vi "Add setting.vi"(7 "setting reference":refnum<vi>, 8 "error in (no error)":errorcluster, 11 "ServiceManager in":refnum<class "ServiceManager.lvclass">) -> (0 "error out":errorcluster, 3 "ServiceManager out":refnum<class "ServiceManager.lvclass">)   [LabVIEW 2012, in "ServiceManager.lvclass"]
uses:
  ServiceManager.lvclass
  settings_cluster.ctl
  Murmex/LabVIEW/Murmex/Murmex/component_specification_cluster.ctl
  ServiceManager.lvclass/ServiceManager.ctl
  Murmex/LabVIEW/Murmex/Murmex/Murmex.lvclass
panel:
  in  "button:cancel":bool
  in  "button:confirm":bool
  in  "Name":string
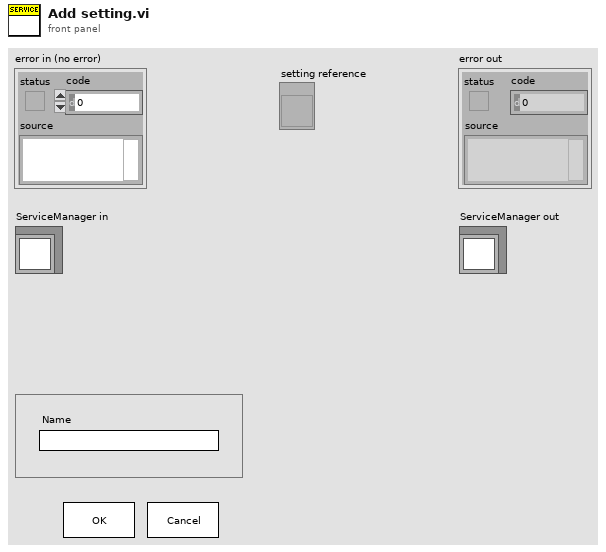
[diagram p1: front panel]
types:
  T1 = typedef "ServiceManager.lvclass/settings_cluster.ctl" = cluster{"components":T2[]}
  T2 = typedef "Murmex.lvlib/Murmex.lvclass/component_specification_cluster.ctl" = cluster{"name":string, "language":string, "host name":string, "id":string}
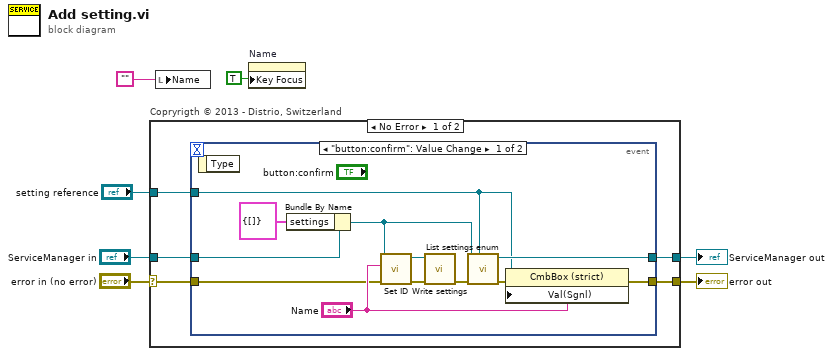
[diagram p0: block diagram]
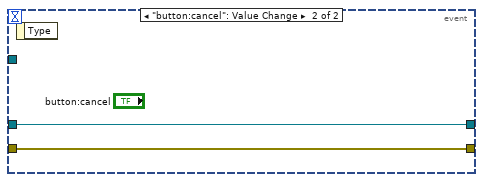
[diagram p2: hidden frame]
diagram:
  n1 = case "Copryrigth © 2013 - Distrio, Switzerland" shown="No Error" "error in (no error)" {
    selector: "error in (no error)" -> [w10 w28]
    tunnel: [w9 w28] -> w6
    tunnel: [w11 w27] -> w4
    tunnel: "ServiceManager in" -> [w12 w27]
    tunnel: "setting reference" -> [w8 _]
    frame No Error {
      n2 = event shown="[0] \"button:confirm\": Value Change" {
        selector: _ -> [_ _]
        dyn-events: _ -> [_ _]
        timeout: _ -> [_ _]
        tunnel: w12 -> [w24 w26]
        tunnel: [w23 w26] -> w11
        tunnel: w10 -> [w16 w25]
        tunnel: [w20 w25] -> w9
        tunnel: w8 -> [w22 _]
        event "button:confirm": Value Change {
          n3 = event-data() -> ()  [unwired: 1 in, 1 out]
          n4 = Bundle By Name(cluster=w24, "settings"=T1 {"components"=[]}) -> (w13:refnum<class "ServiceManager.lvclass">)
          n5 = call "Set ID.vi"("error in (no error)"=w16, "id"="Name", "Murmex in"=w13) -> ("error out"=w15:errorcluster, "Murmex out"=w17:refnum<class "ServiceManager.lvclass">)  [unwired: 7 in]
          n6 = call-dynamic "Write settings.vi"("error in (no error)"=w15, "ServiceManager in"=w17) -> ("error out"=w14:errorcluster)  [unwired: 6 in, 3 out]
          n7 = call-dynamic "List settings enum.vi"("setting enum reference"=w22, "error in (no error)"=w14, "ServiceManager in"=w13) -> ("error out"=w21:errorcluster, "ServiceManager out"=w23:refnum<class "ServiceManager.lvclass">)  [unwired: 7 in]
          n8 = property class="CmbBox (strict)"(reference=w22, error in=w21, "Val(Sgnl)"="Name") -> (error out=w20:errorcluster)  [unwired: 1 out]
        }
        event "button:cancel": Value Change {
          n9 = event-data() -> ()  [unwired: 1 in, 1 out]
        }
      }
    }
    frame Error {
    }
  }
  "error out" <- w6
  "ServiceManager out" <- w4
  n10 = local write "Name"("") -> ()
  n11 = property on="Name" class="Str"("Key Focus"=TRUE) -> ()  [unwired: 2 in, 2 out]
